vi "From JSON.vi"(8 "error in":errorcluster, 10 "JSON":string, 11 "Theme Config in":refnum<class "Theme Config.lvclass">) -> (0 "error out":errorcluster, 3 "Theme Config out":refnum<class "Theme Config.lvclass">)   [LabVIEW 2021, in "Theme Config.lvclass"]
doc: "convert the class data into a json cluster for proper conversion\n\n<b>Code Developed By:</b> +\nDaniel Coons +\nTechnology Service Corporation +\nwww.tsc.com/atcs"
uses:
  Theme Config.lvclass
  Theme Config.lvclass/Theme Config.ctl
  <vilib>/JDP Science/JSONtext/JSONtext.lvlib
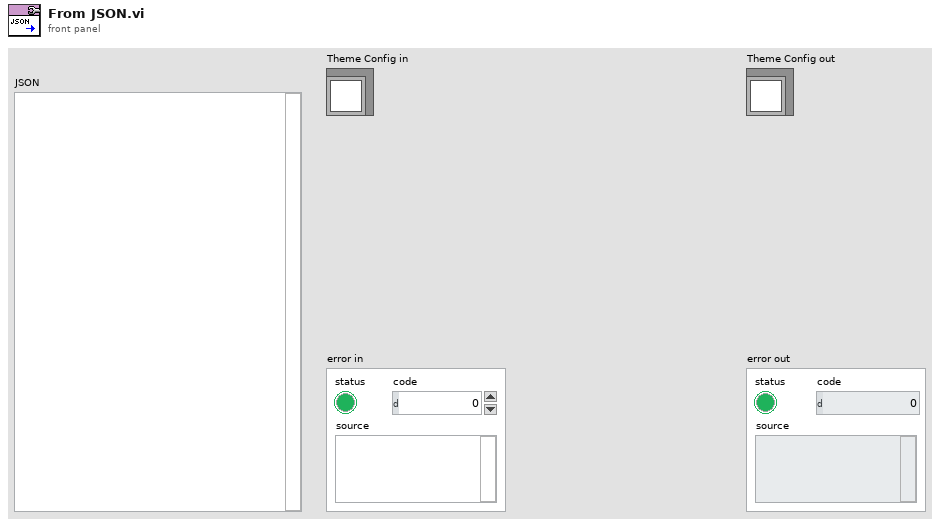
[diagram p1: front panel]
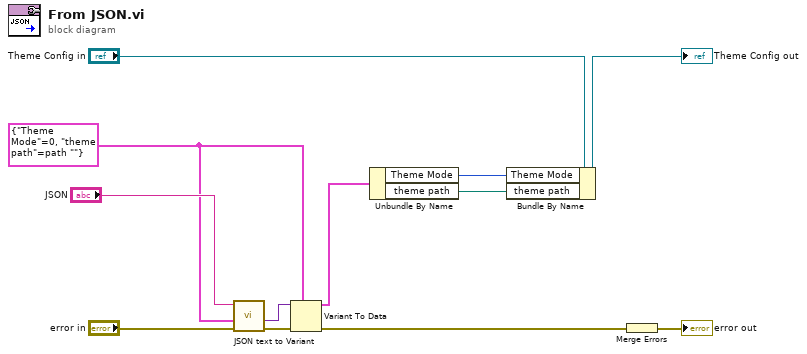
[diagram p0: block diagram]
diagram:
  w3 = cluster{"Theme Mode":u16, "theme path":path} {"Theme Mode"=0, "theme path"=path ""} ("Cluster of class private data")
  n1 = call <vilib>:"JSON text to Variant.vi"("error in (no error)"="error in", "Data Type"=w3, "JSON"="JSON") -> ("error out"=w5:errorcluster, "Variant out"=w4:variant)  [unwired: 7 in]
  n2 = Variant To Data(error in=w5, type=w3, Variant=w4) -> (data=w1:cluster{"Theme Mode":u16, "theme path":path}, error out=w2:errorcluster)
  n3 = Unbundle By Name(w1) -> ("Theme Mode"=w8:u16, "theme path"=w7:path)
  n4 = Bundle By Name(cluster="Theme Config in", "Theme Mode"=w8, "theme path"=w7) -> (→"Theme Config out":refnum<class "Theme Config.lvclass">)
  n5 = Merge Errors(w2) -> (→"error out":errorcluster)
